vi "Write DVR.vi"(8 "error in (no error)":errorcluster, 10 "DVR":refnum<data-value>, 11 "Subject in":refnum<class "Subject.lvclass">) -> (0 "error out":errorcluster, 3 "Subject out":refnum<class "Subject.lvclass">)   [LabVIEW 2012]
uses:
  Subject.lvclass
  Observer/Observer.lvclass
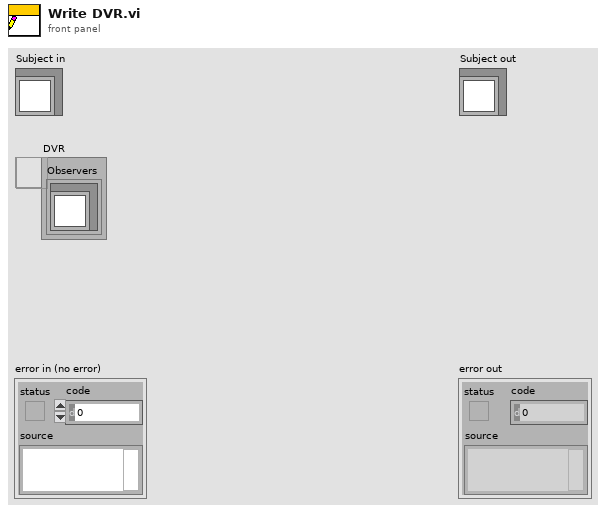
[diagram p1: front panel]
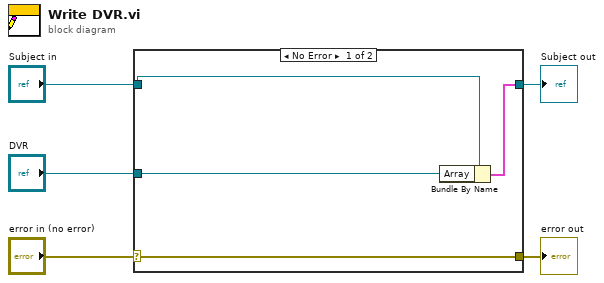
[diagram p0: block diagram]
diagram:
  n1 = case shown="No Error" "error in (no error)" {
    selector: "error in (no error)" -> [w9 w10]
    tunnel: [w9 w10] -> w4
    tunnel: [w7 w11] -> w2
    tunnel: "Subject in" -> [w8 w11]
    tunnel: "DVR" -> [w6 _]
    frame No Error {
      n2 = Bundle By Name(cluster=w8, "Array"=w6) -> (w7:cluster{})
    }
    frame Error {
    }
  }
  "error out" <- w4
  "Subject out" <- w2
